vi "fftw_execute.vi"(8 "error in (no error)":errorcluster, 11 "*plan":u64) -> (0 "error out":errorcluster, 3 "*plan (copy)":u64)   [LabVIEW 2020, in "FFTWDLL.lvlib"]
doc: "Execute FFTW plan."
uses:
  FFTWDLL.lvlib
  dll/libfftw3-3.dll
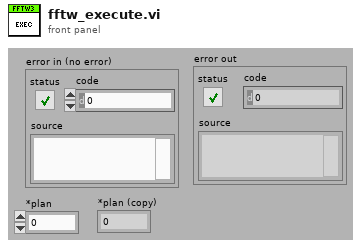
[diagram p1: front panel]
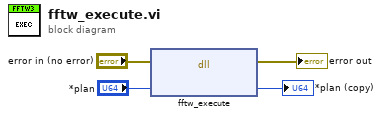
[diagram p0: block diagram]
diagram:
  n1 = dll-call lib="F:/FFTWDLL/dll/libfftw3-3.dll" fn="fftw_execute"(error in="error in (no error)", "*plan"="*plan") -> (error out=→"error out":errorcluster, "*plan"=→"*plan (copy)":u64)  [unwired: 3 in, 1 out]
